vi "CloseCamera.vi"(8 "error in (no error)":errorcluster, 11 "Config In":T1) -> (0 "error out":errorcluster, 3 "Config Out":T1)   [LabVIEW 2019]
uses:
  Settings/Settings.ctl
  Support/Hardware Configuration.ctl
  Support/Camera Configuration.ctl
  E:/DevHardSoftware/MMicroscopy/HardwareAdapter/Camera/Dependencies/PVCamNET.dll
  Dependencies/PVCamNET.dll
  <vilib>/userdefined/High Color/IMAQdx.ctl
  Logging/Logging Configuration.ctl
  controls/UI Configuration.ctl
  Logging/Logging.lvlib
  Settings/Settings.lvlib
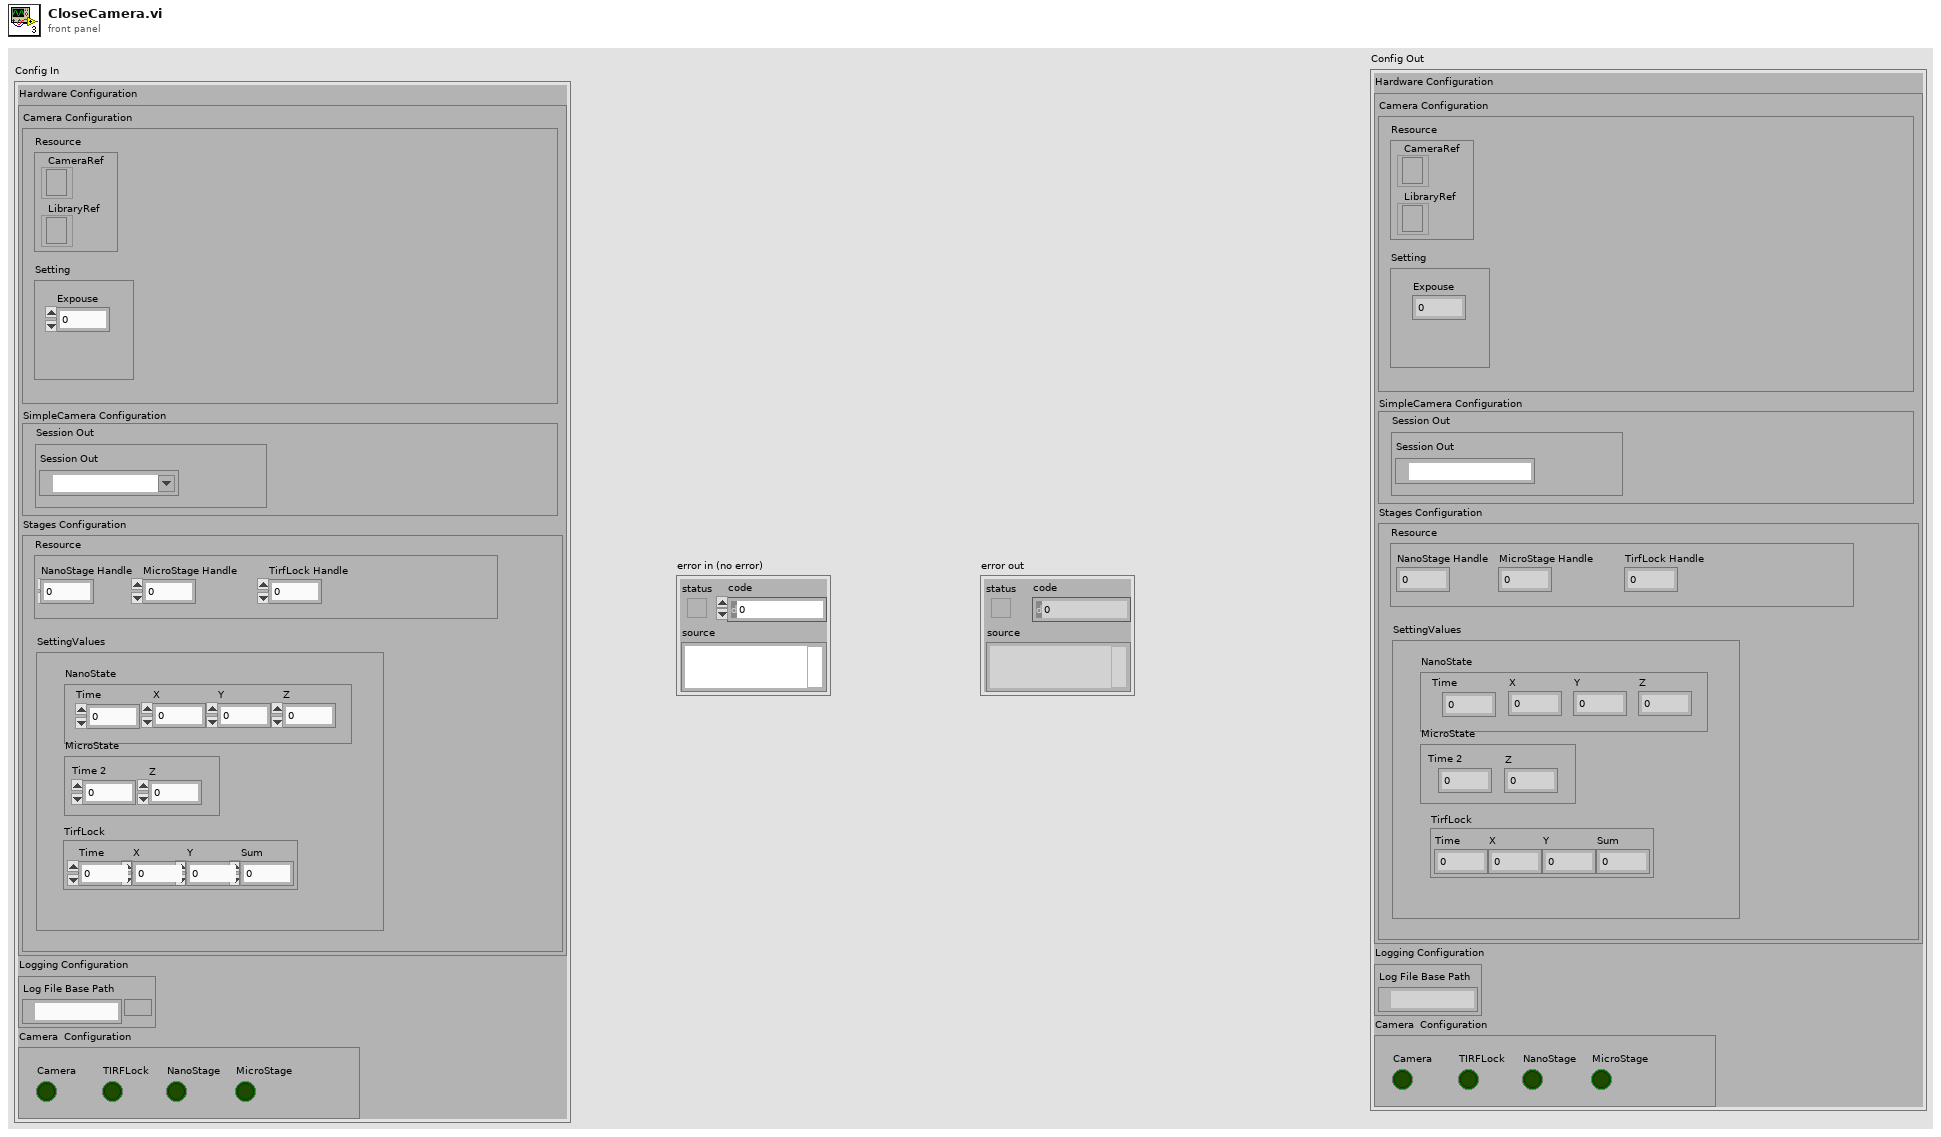
[diagram p1: front panel]
types:
  T1 = typedef "Settings.lvlib/Settings.ctl" = cluster{"Hardware Configuration":T2, "Logging Configuration":T5, "UI Configuration":T6}
  T2 = typedef "Hardware Configuration.ctl" = cluster{"Camera Configuration":T3, "SimpleCamera Configuration":cluster{"Resource":cluster{"Session Out":T4}}, "Stages Configuration":cluster{"Resource":cluster{"NanoStage Handle":i32, "MicroStage Handle":i32, "TirfLock Handle":i32}, "SettingValues":cluster{"NanoState":cluster{"Time":dbl, "X":dbl, "Y":dbl, "Z":dbl}, "MicroState":cluster{"Time 2":dbl, "Z":dbl}, "TirfLock":cluster{"Time":dbl, "X":dbl, "Y":dbl, "Sum":dbl}}}}
  T3 = typedef "Camera Configuration.ctl" = cluster{"Resource":cluster{"CameraRef":refnum<k24>, "LibraryRef":refnum<k24>}, "Setting":cluster{"Expouse":dbl}}
  T4 = typedef "IMAQdx.ctl" = refnum<k21>
  T5 = typedef "Logging.lvlib/Logging Configuration.ctl" = cluster{"Log File Base Path":path}
  T6 = typedef "UI Configuration.ctl" = cluster{"Camera":bool, "NanoStage":bool, "MicroStage":bool, "TIRFLock":bool}
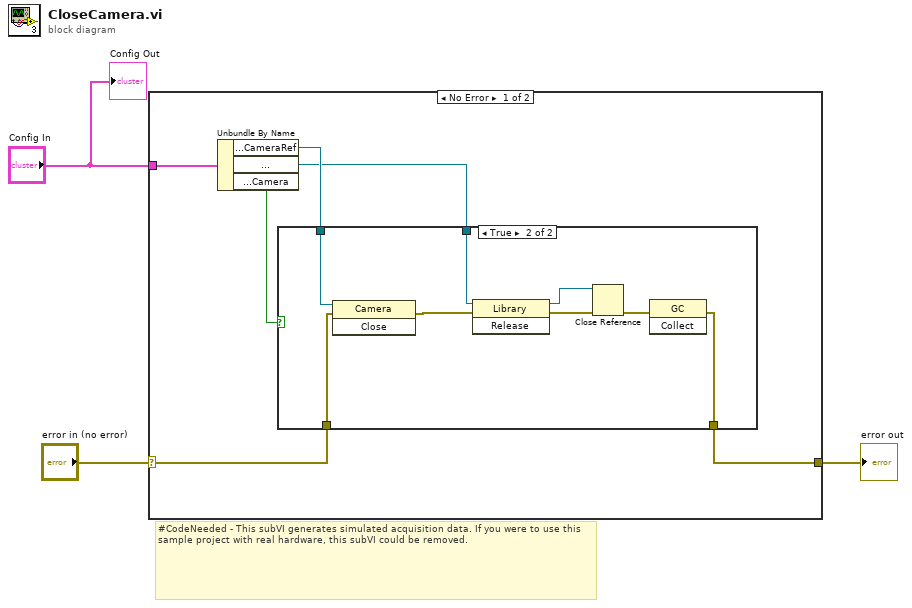
[diagram p0: block diagram]
diagram:
  # "#CodeNeeded - This subVI generates simulated acquisition data. If you were to use this sample project with real hardware, this subVI could be removed."
  n1 = case shown="No Error" "error in (no error)" {
    selector: "error in (no error)" -> [w7 w19]
    tunnel: [w5 w19] -> w2
    tunnel: "Config In" -> [w9 _]
    frame No Error {
      n2 = Unbundle By Name(w9) -> ("Hardware Configuration.Camera Configuration.Resource.CameraRef"=w8:refnum<k24>, "Hardware Configuration.Camera Configuration.Resource.LibraryRef"=w6:refnum<k24>, "UI Configuration.Camera"=w4:bool)
      n3 = case shown="True" w4 {
        tunnel: w8 -> [_ w18]
        tunnel: w7 -> [w10 w17]
        tunnel: w6 -> [_ w14]
        tunnel: [w10 w12] -> w5
        frame False {
        }
        frame True {
          n4 = invoke class="Camera" method="Close"(reference=w18, error in=w17) -> (error out=w16:errorcluster)  [unwired: 1 in, 2 out]
          n5 = invoke class="Library" method="Release"(reference=w14, error in=w16) -> (reference out=w11:refnum<k24>, error out=w15:errorcluster)  [unwired: 1 in, 1 out]
          n6 = Close Reference(reference=w11, error in (no error)=w15) -> (error out=w13:errorcluster)
          n7 = invoke class="GC" method="Collect"(error in=w13) -> (error out=w12:errorcluster)  [unwired: 2 in, 2 out]
        }
      }
    }
    frame Error {
    }
  }
  "error out" <- w2
  "Config Out" <- "Config In"
